vi "Command-RegisterWindow.vi"(8 "error in (no error)":errorcluster, 10 "Data":T1, 11 "Engine in":refnum<class "Engine.lvclass">) -> (0 "error out":errorcluster, 3 "Engine out":refnum<class "Engine.lvclass">)   [LabVIEW 2020, in "GLF.lvlib" / "Engine.lvclass"]
uses:
  Engine.lvclass
  Window/Window.lvclass
  Engine.lvclass/Engine.ctl
  Command-RegisterWindow--cluster.ctl
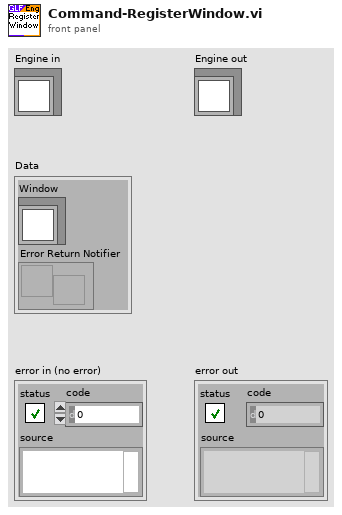
[diagram p1: front panel]
types:
  T1 = typedef "GLF.lvlib/Engine.lvclass/Command-RegisterWindow--cluster.ctl" = cluster{"Window":refnum<class "Window.lvclass">, "Error Return Notifier":refnum<notifier>}
  T2 = typedef "SDL3.lvlib/Video.lvlib/WindowID--integer.ctl" = u32
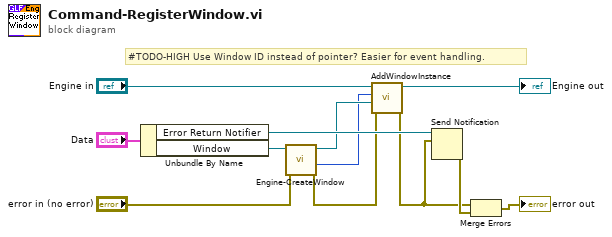
[diagram p0: block diagram]
diagram:
  # "#TODO-HIGH Use Window ID instead of pointer? Easier for event handling."
  n1 = Unbundle By Name("Data") -> ("Error Return Notifier"=w12:refnum<notifier>, "Window"=w10:refnum<class "Window.lvclass">)
  n2 = call "Engine-CreateWindow.vi"("error in (no error)"="error in (no error)", "Window in"=w10) -> ("error out"=w3:errorcluster, "Window ID"=w1:T2, "Window out"=w5:refnum<class "Window.lvclass">)  [unwired: 6 in, 1 out]
  n3 = call "AddWindowInstance.vi"("error in (no error)"=w3, "Window Instance"=w5, "Window ID"=w1, "Engine in"="Engine in") -> ("error out"=w2:errorcluster, "Engine out"=→"Engine out":refnum<class "Engine.lvclass">)  [unwired: 6 in]
  n4 = Send Notification(notification=w2, notifier=w12) -> (error out=w11:errorcluster)  [unwired: 1 in, 1 out]
  n5 = Merge Errors(w2, w11) -> (→"error out":errorcluster)
